vi "hmi_dialog_text_box.vi"(7 "vi_reference":refnum<vi>, 8 "error in (no error)":errorcluster, 9 "vi_maximums":T1={"max_height"=102, "max_width"=300, "control_height"=50, "control_width"=24}, 11 "dialog_text in":string) -> (0 "error out":errorcluster, 2 "enable_scrollbar":bool, 3 "dialog_text out":string)   [LabVIEW 2015, in "lv-dialog-interfaces.lvlib"]
doc: "This can be used to re-size the size of the front panel depending on the text."
uses:
  lv-dialog-interfaces.lvlib
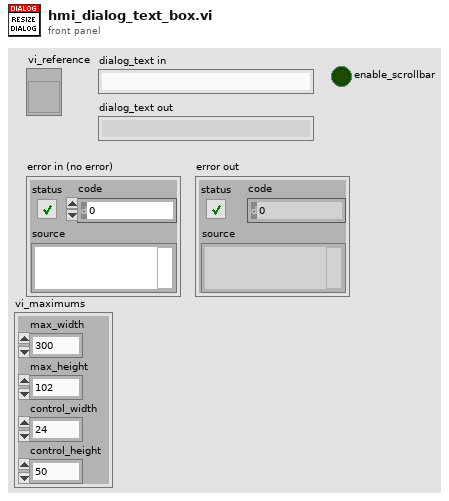
[diagram p1: front panel]
types:
  T1 = cluster{"max_height":i16, "max_width":i16, "control_height":i16, "control_width":i16}
  T2 = typedef "LVRectTypeDef.ctl" = cluster{"Left":i16, "Top":i16, "Right":i16, "Bottom":i16}
  T3 = cluster{"left":i16, "top":i16, "right":i16, "bottom":i16}
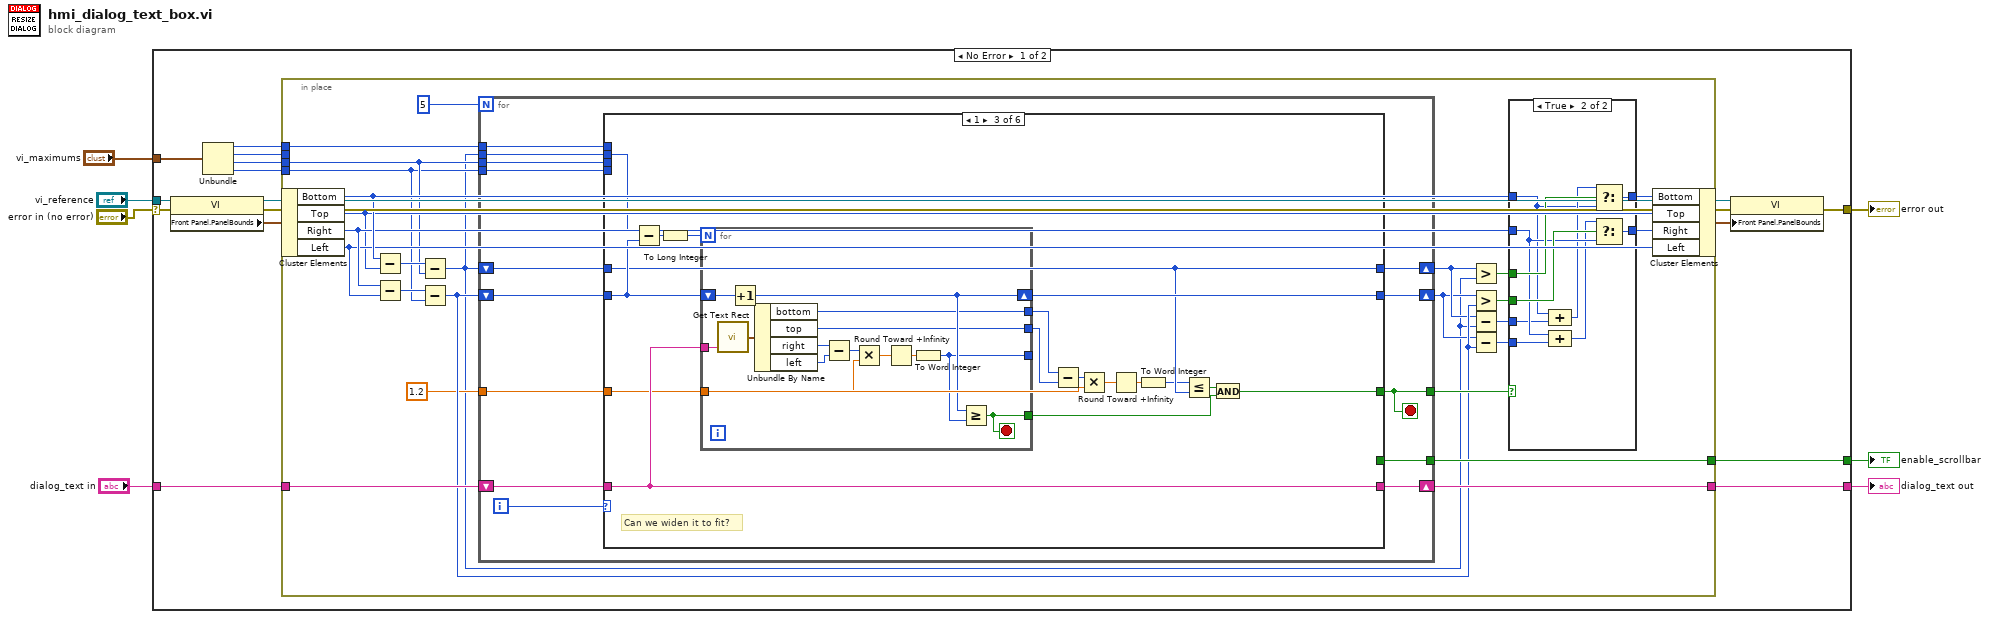
[diagram p0: block diagram]
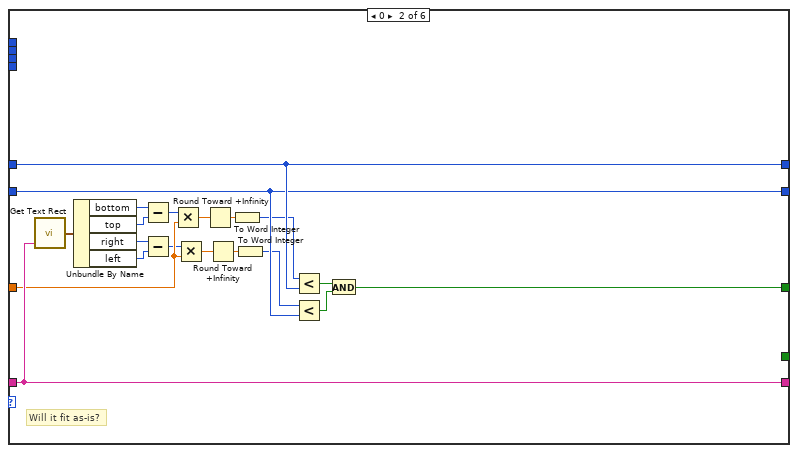
[diagram p3: hidden frame]
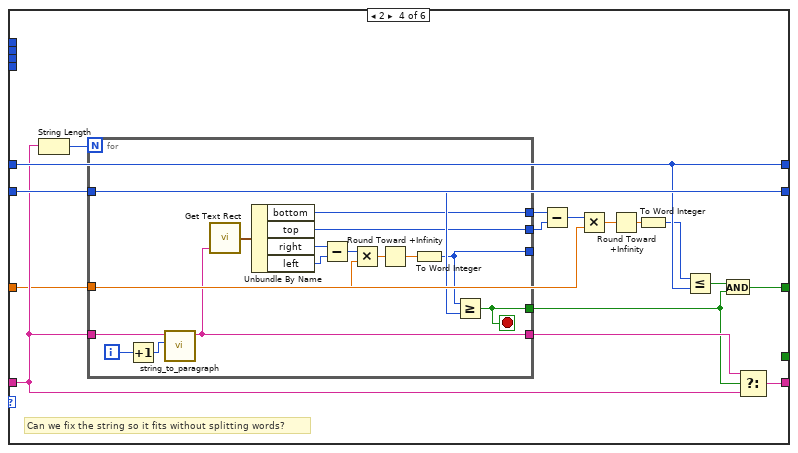
[diagram p4: hidden frame]
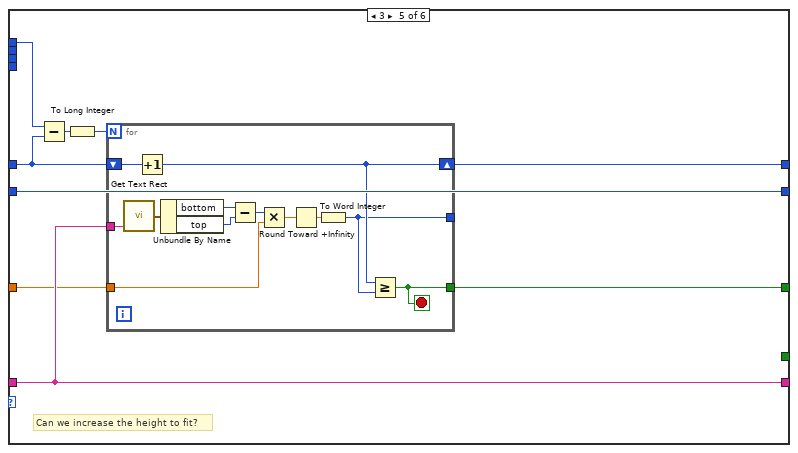
[diagram p5: hidden frame]
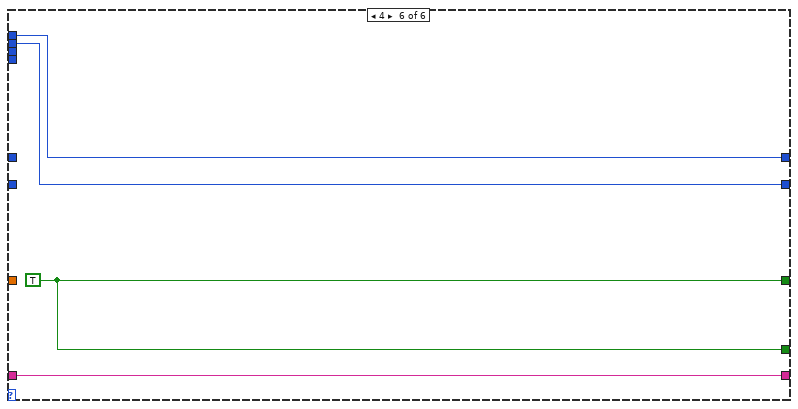
[diagram p6: hidden frame]
diagram:
  n1 = case shown="No Error" "error in (no error)" {
    selector: "error in (no error)" -> [w17 w185]
    tunnel: "vi_reference" -> [w18 _]
    tunnel: [w8 w185] -> w5
    tunnel: "dialog_text in" -> [w16 w186]
    tunnel: [w15 _] -> w3
    tunnel: [w14 w186] -> w2
    tunnel: "vi_maximums" -> [w13 _]
    frame No Error {
      n2 = property class="VI"(reference=w18, error in=w17) -> (reference out=w19:refnum<vi>, error out=w20:errorcluster, "Front Panel.PanelBounds"=w21:T2)
      n3 = Unbundle(w13) -> ("max_height"=w12:i16, "max_width"=w11:i16, "control_height"=w10:i16, "control_width"=w9:i16)
      n4 = in-place {
        in-place-border: w10 -> [w29]
        in-place-border: w9 -> [w28]
        in-place-border: w12 -> [w32]
        in-place-border: w11 -> [_]
        in-place-border: w16 -> [w39]
        in-place-border: [w37] -> w15
        in-place-border: [w36] -> w14
        n5 = in-place-cluster #1(w21) -> ("Bottom"=w47:i16, "Top"=w42:i16, "Right"=w44:i16, "Left"=w43:i16)
        n6 = Subtract(x=w47, y=w42) -> (x-y=w34:i16)
        n7 = Subtract(x=w44, y=w43) -> (x-y=w33:i16)
        n8 = Subtract(x=w34, y=w29) -> (x-y=w23:i16)
        n9 = Subtract(x=w33, y=w28) -> (x-y=w31:i16)
        n10 = for {
          N: 5 -> [_]
          shift-right: [w55] -> w27
          shift-left: w23 -> [w59]
          shift-right: [w54] -> w26
          shift-left: w31 -> [w58]
          tunnel: w23 -> [w57]
          tunnel: w32 -> [w56]
          shift-right: [w53] -> w36
          shift-left: w39 -> [w61]
          tunnel: [w52] -> w37
          tunnel: [w51] -> w35
          tunnel: 1.2 ("y") -> [w50]
          tunnel: w29 -> [w49]
          tunnel: w28 -> [w48]
          i -> [w60]
          stop <- w51 stop-if-true
          n11 = case shown="1" w60 {
            tunnel: w61 -> [w62 w74 w97 w124 w154 w172]
            tunnel: w59 -> [w64 w76 w90 w129 w151 _]
            tunnel: w58 -> [w63 w75 w99 w131 w150 _]
            tunnel: w57 -> [_ _ w100 _ _ w170]
            tunnel: w56 -> [_ _ _ _ w155 w169]
            tunnel: [w64 w76 w90 w129 w149 w169] -> w55
            tunnel: [w63 w75 w101 w131 w150 w170] -> w54
            tunnel: [_ w77 w91 w125 w152 w171] -> w51
            tunnel: [w62 w74 w97 w123 w154 w172] -> w53
            tunnel: [_ _ _ _ _ w171] -> w52
            tunnel: w50 -> [_ w69 w85 w116 w148 _]
            tunnel: w49 -> [_ _ _ _ _ _]
            tunnel: w48 -> [_ _ _ _ _ _]
            frame Default {
            }
            frame 0 {
              # "Will it fit as-is?"
              n12 = call <vilib>:"Get Text Rect.vi"("text"=w74) -> ("rect"=w84:T3)  [unwired: 8 in]
              n13 = Unbundle By Name(w84) -> ("bottom"=w83:i16, "top"=w82:i16, "right"=w81:i16, "left"=w80:i16)
              n14 = Subtract(x=w83, y=w82) -> (x-y=w68:i16)
              n15 = Subtract(x=w81, y=w80) -> (x-y=w66:i16)
              n16 = Multiply(x=w68, y=w69) -> (x*y=w72:dbl)
              n17 = Multiply(x=w66, y=w69) -> (x*y=w71:dbl)
              n18 = Round Toward +Infinity(x=w72) -> (ceil(x): smallest int >= x=w73:dbl)
              n19 = Round Toward +Infinity(x=w71) -> (ceil(x): smallest int >= x=w70:dbl)
              n20 = To Word Integer(number=w73) -> (16bit integer=w67:i16)
              n21 = To Word Integer(number=w70) -> (16bit integer=w65:i16)
              n22 = Less?(x=w67, y=w76) -> (x < y?=w79:bool)
              n23 = Less?(x=w65, y=w75) -> (x < y?=w78:bool)
              n24 = And(x=w79, y=w78) -> (x .and. y?=w77:bool)
            }
            frame 1 {
              # "Can we widen it to fit?"
              n25 = Subtract(x=w100, y=w99) -> (x-y=w98:i16)
              n26 = To Long Integer(number=w98) -> (32bit integer=w96:i32)
              n27 = for {
                N: w96 -> [_]
                tunnel: [w102] -> _
                tunnel: [w109] -> w92
                tunnel: w97 -> [w110]
                shift-right: [w111] -> w101
                shift-left: w99 -> [w112]
                tunnel: [w108] -> w95
                tunnel: [w107] -> w94
                tunnel: w85 -> [w103]
                stop <- w109 stop-if-true
                n28 = call <vilib>:"Get Text Rect.vi"("text"=w110) -> ("rect"=w115:T3)  [unwired: 8 in]
                n29 = Increment(x=w112) -> (x+1=w111:i16)
                n30 = Unbundle By Name(w115) -> ("bottom"=w108:i16, "top"=w107:i16, "right"=w114:i16, "left"=w113:i16)
                n31 = Subtract(x=w114, y=w113) -> (x-y=w104:i16)
                n32 = Multiply(x=w104, y=w103) -> (x*y=w105:dbl)
                n33 = Round Toward +Infinity(x=w105) -> (ceil(x): smallest int >= x=w106:dbl)
                n34 = To Word Integer(number=w106) -> (16bit integer=w102:i16)
                n35 = Greater Or Equal?(x=w111, y=w102) -> (x >= y?=w109:bool)
              }
              n36 = Subtract(x=w95, y=w94) -> (x-y=w87:i16)
              n37 = Multiply(x=w87, y=w85) -> (x*y=w88:dbl)
              n38 = Round Toward +Infinity(x=w88) -> (ceil(x): smallest int >= x=w89:dbl)
              n39 = To Word Integer(number=w89) -> (16bit integer=w86:i16)
              n40 = Less Or Equal?(x=w86, y=w90) -> (x <= y?=w93:bool)
              n41 = And(x=w93, y=w92) -> (x .and. y?=w91:bool)
            }
            frame 2 {
              # "Can we fix the string so it fits without splitting words?"
              n42 = String Length(string=w124) -> (length=w130:i32)
              n43 = for {
                N: w130 -> [_]
                tunnel: w124 -> [w141]
                tunnel: w131 -> [w143]
                tunnel: [w140] -> w121
                tunnel: [w139] -> w127
                tunnel: [w138] -> w126
                tunnel: [w137] -> w122
                tunnel: [w133] -> _
                tunnel: w116 -> [w132]
                i -> [w147]
                stop <- w140 stop-if-true
                n44 = Increment(x=w147) -> (x+1=w142:i32)
                n45 = call "string_to_paragraph.vi"("no_of_char"=w142, "string in"=w141) -> ("string out"=w137:string)  [unwired: 8 in, 1 out]
                n46 = call <vilib>:"Get Text Rect.vi"("text"=w137) -> ("rect"=w144:T3)  [unwired: 8 in]
                n47 = Unbundle By Name(w144) -> ("bottom"=w139:i16, "top"=w138:i16, "right"=w145:i16, "left"=w146:i16)
                n48 = Subtract(x=w145, y=w146) -> (x-y=w134:i16)
                n49 = Multiply(x=w134, y=w132) -> (x*y=w135:dbl)
                n50 = Round Toward +Infinity(x=w135) -> (ceil(x): smallest int >= x=w136:dbl)
                n51 = To Word Integer(number=w136) -> (16bit integer=w133:i16)
                n52 = Greater Or Equal?(x=w133, y=w143) -> (x >= y?=w140:bool)
              }
              n53 = Subtract(x=w127, y=w126) -> (x-y=w118:i16)
              n54 = Multiply(x=w118, y=w116) -> (x*y=w119:dbl)
              n55 = Round Toward +Infinity(x=w119) -> (ceil(x): smallest int >= x=w120:dbl)
              n56 = To Word Integer(number=w120) -> (16bit integer=w117:i16)
              n57 = Less Or Equal?(x=w117, y=w129) -> (x <= y?=w128:bool)
              n58 = And(x=w128, y=w121) -> (x .and. y?=w125:bool)
              n59 = Select(t=w122, s=w121, f=w124) -> (s? t:f=w123:string)
            }
            frame 3 {
              # "Can we increase the height to fit?"
              n60 = Subtract(x=w155, y=w151) -> (x-y=w156:i16)
              n61 = To Long Integer(number=w156) -> (32bit integer=w153:i32)
              n62 = for {
                N: w153 -> [_]
                tunnel: [w166] -> w152
                tunnel: w154 -> [w167]
                shift-right: [w162] -> w149
                shift-left: w151 -> [w163]
                tunnel: [w157] -> _
                tunnel: w148 -> [w159]
                stop <- w166 stop-if-true
                n63 = call <vilib>:"Get Text Rect.vi"("text"=w167) -> ("rect"=w168:T3)  [unwired: 8 in]
                n64 = Increment(x=w163) -> (x+1=w162:i16)
                n65 = Unbundle By Name(w168) -> ("bottom"=w165:i16, "top"=w164:i16)
                n66 = Subtract(x=w165, y=w164) -> (x-y=w158:i16)
                n67 = Multiply(x=w158, y=w159) -> (x*y=w160:dbl)
                n68 = Round Toward +Infinity(x=w160) -> (ceil(x): smallest int >= x=w161:dbl)
                n69 = To Word Integer(number=w161) -> (16bit integer=w157:i16)
                n70 = Greater Or Equal?(x=w162, y=w157) -> (x >= y?=w166:bool)
              }
            }
            frame 4 {
              w171 = TRUE
            }
          }
        }
        n71 = Greater?(x=w27, y=w23) -> (0:w41:bool)
        n72 = Greater?(x=w26, y=w31) -> (0:w40:bool)
        n73 = Subtract(x=w27, y=w23) -> (x-y=w24:i16)
        n74 = Subtract(x=w26, y=w31) -> (x-y=w25:i16)
        n75 = case shown="True" w35 {
          tunnel: w47 -> [w174 w178]
          tunnel: [w174 w177] -> w46
          tunnel: w24 -> [_ w175]
          tunnel: w44 -> [w173 w182]
          tunnel: [w173 w179] -> w45
          tunnel: w25 -> [_ w176]
          tunnel: w41 -> [_ w184]
          tunnel: w40 -> [_ w183]
          frame False {
          }
          frame True {
            n76 = Compound Arithmetic op=ADD(w178, w175) -> (w180:i16)
            n77 = Compound Arithmetic op=ADD(w182, w176) -> (w181:i16)
            n78 = Select(t=w180, s=w184, f=w178) -> (s? t:f=w177:i16)
            n79 = Select(t=w181, s=w183, f=w182) -> (s? t:f=w179:i16)
          }
        }
        n80 = in-place-cluster #1("Bottom"=w46, "Top"=w42, "Right"=w45, "Left"=w43) -> (w22:T2)
      }
      n81 = property class="VI"(reference=w19, error in=w20, "Front Panel.PanelBounds"=w22) -> (error out=w8:errorcluster)  [unwired: 1 out]
    }
    frame Error {
    }
  }
  "error out" <- w5
  "enable_scrollbar" <- w3
  "dialog_text out" <- w2
